vi "05b-multiple_functions.vi"() -> ()   [LabVIEW 2018, in "LV2Julia_examples.lvlib"]
uses:
  LV2Julia_examples.lvlib
  LV2Julia_core/VIs/Server or client state.ctl
  LV2Julia_core/VIs/detailed error info.ctl
  LV2Julia_core/VIs/StackFrame.ctl
  LV2Julia_core/VIs/Commands.ctl
  b50b62fa-0ed7-4d6a-8a9d-aa54acf293b0.vi
  b50b62fa-0ed7-4d6a-8a9d-aa54acf293b0.vi/b0ffba6b-3b8e-4ae7-8fb7-95bf2cbab623.vi
  b50b62fa-0ed7-4d6a-8a9d-aa54acf293b0.vi/b0ffba6b-3b8e-4ae7-8fb7-95bf2cbab623.vi/b7d17f2f-a16a-42de-b47e-6859e258df3c.vi
  b50b62fa-0ed7-4d6a-8a9d-aa54acf293b0.vi/b0ffba6b-3b8e-4ae7-8fb7-95bf2cbab623.vi/d3f2d99f-4af2-4ced-bf3b-fac587840905.vi
  b50b62fa-0ed7-4d6a-8a9d-aa54acf293b0.vi/b0ffba6b-3b8e-4ae7-8fb7-95bf2cbab623.vi/9c852c56-c8b0-4d48-a412-f129579acc54.vi
  LV2Julia_core/VIs/jl-scripts path.vi
  LV2Julia_core/VIs/check ID validity.vi
  LV2Julia_core/VIs/bindata_descr to JSON.vi
  LV2Julia_core/VIs/check cluster field names.vi
  LV2Julia_core/VIs/concat JSON.vi
  LV2Julia_core/VIs/build request.vi
  LV2Julia_core/VIs/Parse server response.vi
  LV2Julia_core/VIs/log jl exceptions.vi
  LV2Julia_core/LV2Julia_core.lvlib
panel:
  in  "operation":u16(ring) items=["addition", "subtraction", "multiplication", "division", "conquer"]
  in  "operands":cluster{"x":dbl, "y":dbl}={"x"=2.0, "y"=2.0}
  in  "next":bool
  out "result":dbl=nan
  out "detailed error info":T1
  out "current error":errorcluster
  out "final error":errorcluster
  out "short err code":u8
  in  "stop":bool
  out "ZMQ timeout":bool
  out "Julia script file path":path
  out "temporary script path":path
  out "Jl Server state":T3
  # "available functions loaded on start from the Julia server"
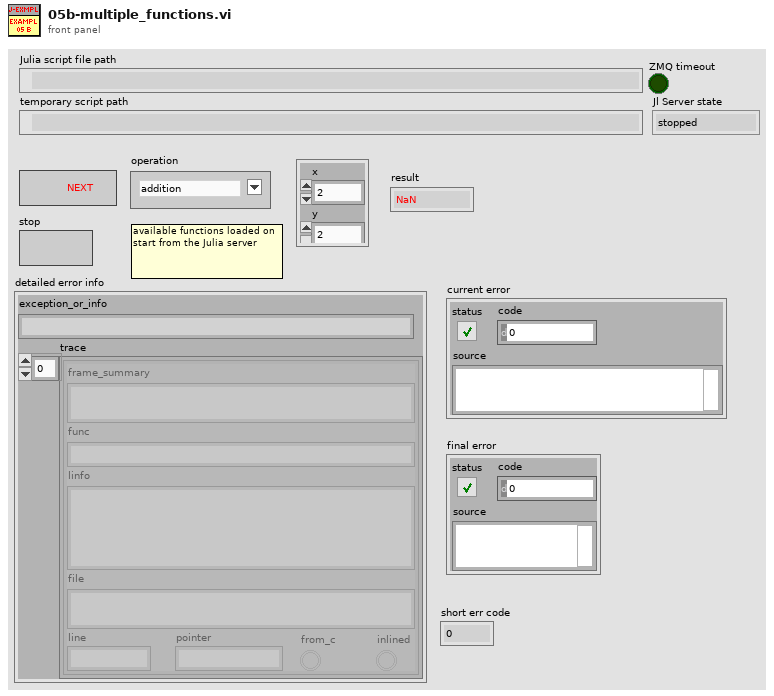
[diagram p1: front panel]
types:
  T1 = typedef "LV2Julia_core.lvlib/detailed error info.ctl" = cluster{"exception_or_info":string, "trace":T2[]}
  T2 = typedef "LV2Julia_core.lvlib/StackFrame.ctl" = cluster{"frame_summary":string, "func":string, "linfo":string, "file":string, "line":i32, "pointer":u64, "from_c":bool, "inlined":bool}
  T3 = typedef "LV2Julia_core.lvlib/Server or client state.ctl" = enum16{"stopped", "running", "unknown"}
  T4 = typedef "LV2Julia_core.lvlib/Commands.ctl" = enum16{"Start Jl-server & Init LV-client", "Send request & Get response ", "Stop Jl-server & Cleanup LV-client", "Cleanup LV-client", "Start Jl-server", "Stop Jl-server", "Init LV-Client", "Cleanup LV-Client", "(not allowed)", "Set LV Client state", "Set Jl Server state", "set ZMQ timeout", "read ZMQ timeout", "read-out state"}
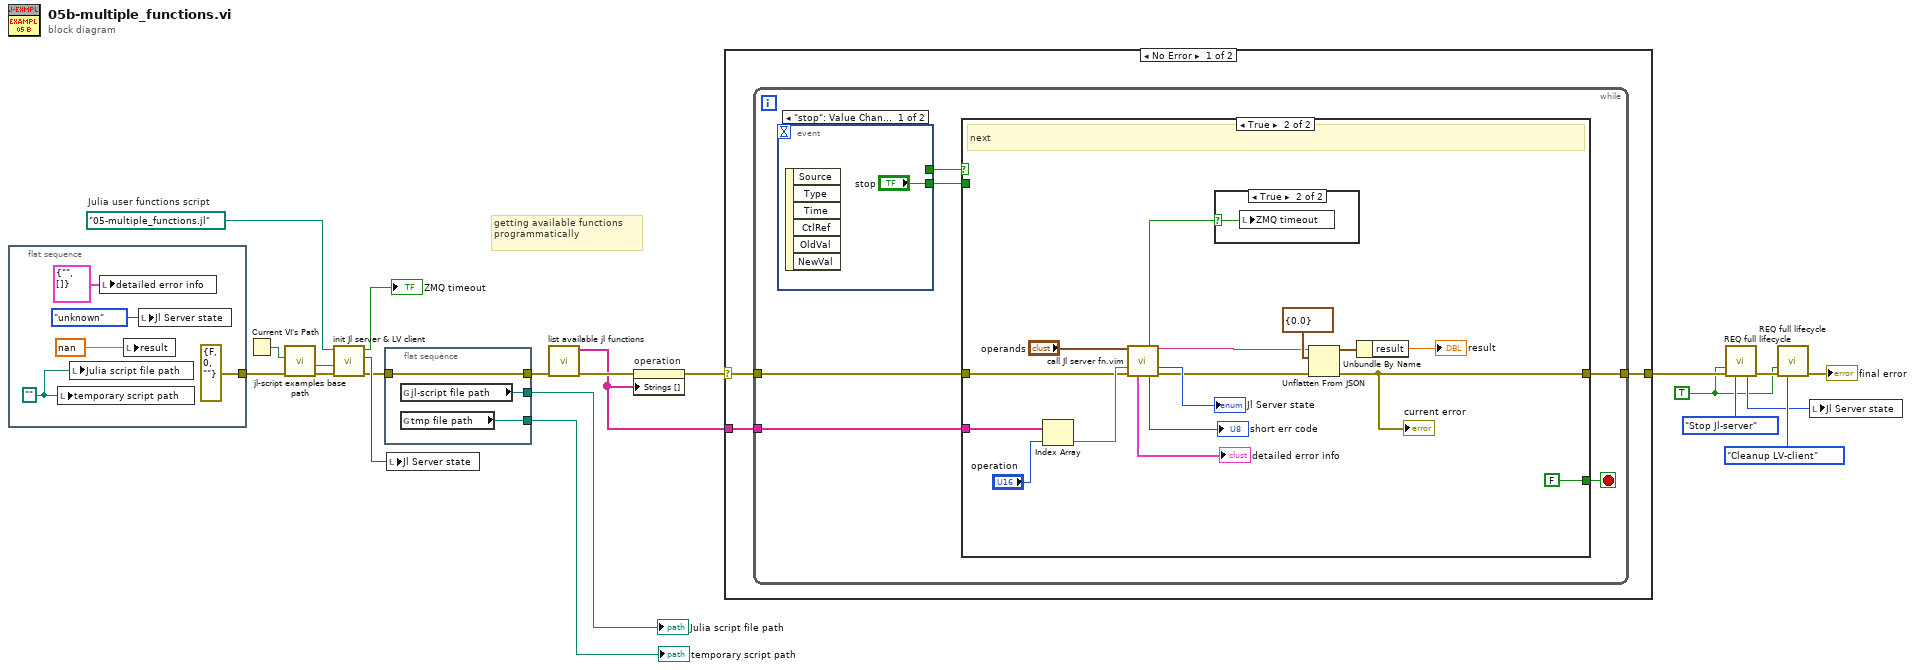
[diagram p0: block diagram]
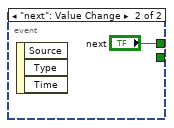
[diagram p2: hidden frame]
diagram:
  w8 = path "05-multiple_functions.jl"  # Julia user functions script
  w13 = TRUE ("Force command")
  # "getting available functions programmatically"
  n1 = flat-sequence {
    tunnel: [errorcluster {"status"=FALSE, "code"=0, "source"=""} ("error in (no error)")] -> w2
    frame #0 {
      w22 = path ""
      n2 = local write "temporary script path"(w22) -> ()
      n3 = local write "Julia script file path"(w22) -> ()
      n4 = local write "detailed error info"(T1 {"exception_or_info"="", "trace"=[]} ("detailed error info")) -> ()
      n5 = local write "result"(nan ("Server response")) -> ()
      n6 = local write "Jl Server state"(Server_or_client_state."unknown" ("Jl Server state out")) -> ()
    }
  }
  n7 = Current VI's Path() -> (path=w4:path)
  n8 = call "jl-script examples base path.vi"("error in (no error)"=w2, "calling example VI path"=w4) -> ("error out"=w3:errorcluster, "jl-script-examples base path"=w1:path)  [unwired: 8 in]
  n9 = call "init Jl server & LV client.vi"("error in (no error)"=w3, "Base path (not a path)"=w1, "Julia user functions script"=w8) -> ("error out"=w5:errorcluster, "Jl Server state out"=w6:T3, "timeout?"=→"ZMQ timeout":bool)  [unwired: 6 in]
  n10 = flat-sequence {
    tunnel: [w29] -> w12
    tunnel: w5 -> [w29]
    tunnel: [w28] -> w15
    tunnel: [w27] -> w16
    frame #0 {
      n11 = global read "jl-scripts path.vi" "jl-script file path"() -> (w28:path)
      n12 = global read "jl-scripts path.vi" "tmp file path"() -> (w27:path)
    }
  }
  n13 = local write "Jl Server state"(w6) -> ()
  n14 = call "list available jl functions.vi"("error in (no error)"=w12) -> ("error out"=w11:errorcluster, "ext_fns"=w9:string[])  [unwired: 5 in, 4 out]
  n15 = property on="operation" class="Ring (strict)"(error in=w11, "Strings []"=w9) -> (error out=w10:errorcluster)  [unwired: 1 in, 1 out]
  n16 = case shown="No Error" w10 {
    selector: w10 -> [w31 w60]
    tunnel: [w32 w60] -> w21
    tunnel: w9 -> [w30 _]
    frame No Error {
      n17 = while {
        tunnel: w31 -> [w37]
        tunnel: [w38] -> w32
        tunnel: w30 -> [w33]
        stop <- w35 stop-if-true
        n18 = event shown="[0] \"stop\": Value Change" {
          selector: _ -> [_ _]
          dyn-events: _ -> [_ _]
          timeout: _ -> [_ _]
          tunnel: [_ "next"] -> w36
          tunnel: ["stop" _] -> w34
          event "stop": Value Change {
            n19 = event-data() -> ()  [unwired: 1 in, 6 out]
          }
          event "next": Value Change {
            n20 = event-data() -> ()  [unwired: 1 in, 3 out]
          }
        }
        n21 = case shown="True" w36 {
          tunnel: [w42 w55] -> w38
          tunnel: w37 -> [w42 w49]
          tunnel: [w41 FALSE ("stop this VI only")] -> w35
          tunnel: w34 -> [w41 _]
          tunnel: w33 -> [_ w53]
          frame False {
            # "stop"
          }
          frame True {
            # "next"
            n22 = Index Array(array=w53, index="operation") -> (element=w50:string)
            n23 = call "call Jl server fn.vim"("Arguments 1"="operands", "fun2call"=w50, "error in (no error)"=w49) -> ("timeout?"=w46:bool, "JSON received"=w44:string, "Jl Server state out"=→"Jl Server state":T3, "detailed error info"=→"detailed error info":T1, "return code"=→"short err code":u8, "error out"=w47:errorcluster)  [unwired: 6 in, 1 out]
            n24 = case shown="True" w46 {
              selector: w46 -> [_ w59]
              frame False {
              }
              frame True {
                n25 = local write "ZMQ timeout"(w59) -> ()
              }
            }
            n26 = Unflatten From JSON(JSON string=w44, type and defaults=cluster{"result":dbl} {"result"=0.0} ("parsed response"), error in (no error)=w47) -> (value=w57:cluster{"result":dbl}, error out=w55:errorcluster)  [unwired: 4 in]
            "current error" <- w55
            n27 = Unbundle By Name(w57) -> ("result"=→"result":dbl)
          }
        }
      }
    }
    frame Error {
    }
  }
  n28 = call "REQ full lifecycle.vi"("Force command"=w13, "error in"=w21, "command"=Commands."Stop Jl-server") -> ("Jl Server state out"=w14:T3, "error out"=w19:errorcluster)  [unwired: 6 in, 5 out]
  n29 = call "REQ full lifecycle.vi"("Force command"=w13, "error in"=w19, "command"=Commands."Cleanup LV-client") -> ("error out"=→"final error":errorcluster)  [unwired: 6 in, 6 out]
  n30 = local write "Jl Server state"(w14) -> ()
  "temporary script path" <- w16
  "Julia script file path" <- w15
